vi "StringsArrayToDotsSeparatedString.vi"(11 "StringArray":string[](array[string])) -> (3 "DotSeparatedString":string)   [LabVIEW 2013, in "Highland T564 DDG.lvclass"]
uses:
  Highland T564 DDG.lvclass
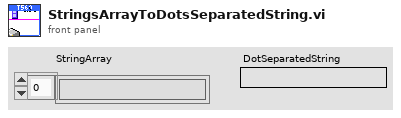
[diagram p1: front panel]
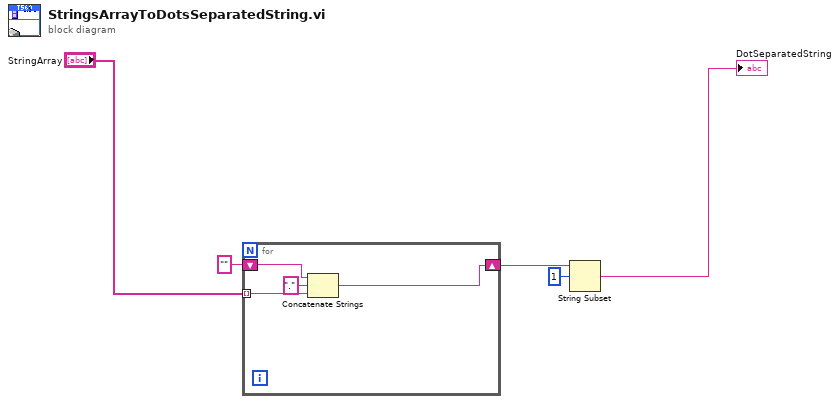
[diagram p0: block diagram]
diagram:
  n1 = for {
    tunnel: "StringArray" -> [w8] mode=indexing
    shift-right: [w6] -> w2
    shift-left: "" -> [w9]
    n2 = Concatenate Strings(w9, "." ("string"), w8) -> (w6:string)
  }
  n3 = String Subset(string=w2, offset (0)=1) -> (substring=→"DotSeparatedString":string)  [unwired: 1 in]
